vi "DPO_7K_Acquisition Mode.vi"(8 "Error In":errorcluster, 9 "Mode":u16(ring) items=["Continuous", "Single"], 10 "Action":u16(ring) items=["Run", "Stop"], 11 "VISA resource name in":refnum<visa-resource-name>) -> (0 "Error Out":errorcluster, 3 "VISA resource name out":refnum<visa-resource-name>)   [LabVIEW 2020]
panel:
  # "RUN/MODE SETTINGS"
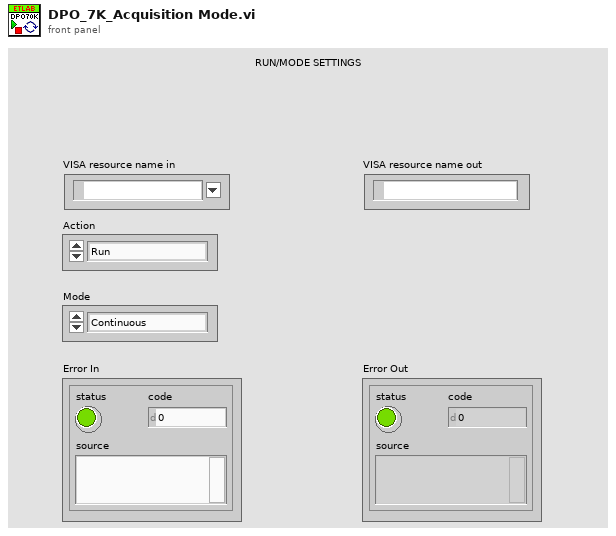
[diagram p1: front panel]
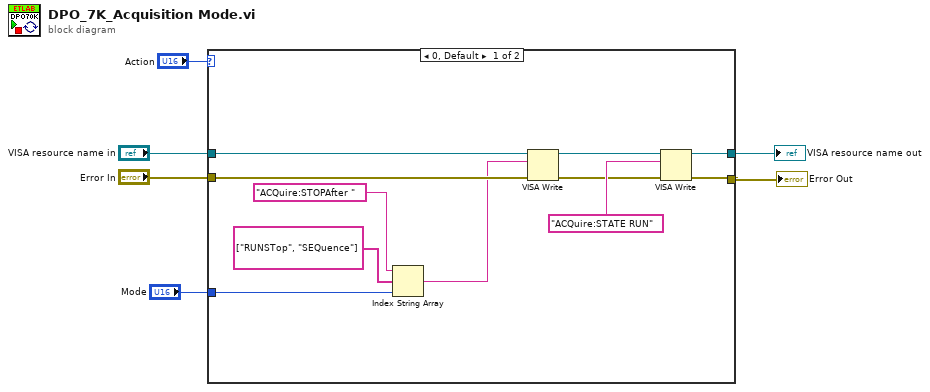
[diagram p0: block diagram]
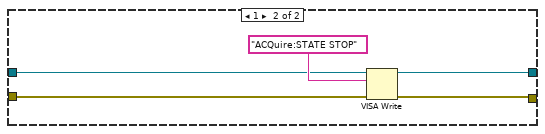
[diagram p2: hidden frame]
diagram:
  n1 = case shown="0, Default" "Action" {
    tunnel: [w14 w18] -> w2
    tunnel: [w13 w19] -> w1
    tunnel: "VISA resource name in" -> [w11 w21]
    tunnel: "Error In" -> [w12 w20]
    tunnel: "Mode" -> [w8 _]
    frame 0, Default {
      n2 = Index String Array(1:w8, 2:string[] ["RUNSTop", "SEQuence"], 3:"ACQuire:STOPAfter ") -> (0:w7:string)
      n3 = VISA Write(VISA resource name=w11, write buffer=w7, error in (no error)=w12) -> (VISA resource name out=w15:refnum<visa-resource-name>, error out=w16:errorcluster)  [unwired: 1 out]
      n4 = VISA Write(VISA resource name=w15, write buffer="ACQuire:STATE RUN", error in (no error)=w16) -> (VISA resource name out=w14:refnum<visa-resource-name>, error out=w13:errorcluster)  [unwired: 1 out]
    }
    frame 1 {
      n5 = VISA Write(VISA resource name=w21, write buffer="ACQuire:STATE STOP", error in (no error)=w20) -> (VISA resource name out=w18:refnum<visa-resource-name>, error out=w19:errorcluster)  [unwired: 1 out]
    }
  }
  "VISA resource name out" <- w2
  "Error Out" <- w1
